vi "20211022_HW02.vi"() -> ()   [LabVIEW 2019]
panel:
  out "Result":string
  in  "N5":i32
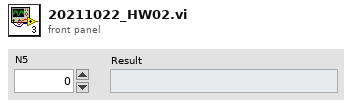
[diagram p1: front panel]
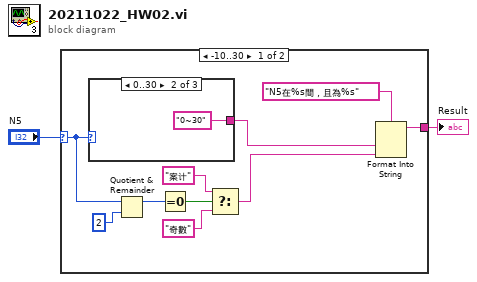
[diagram p0: block diagram]
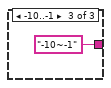
[diagram p3: hidden frame]
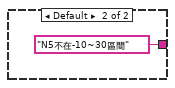
[diagram p4: hidden frame]
diagram:
  n1 = case shown="-10..30" "N5" {
    selector: "N5" -> [w12 _]
    tunnel: [w3 "N5不在-10~30區間"] -> w1
    frame -10..30 {
      n2 = case shown="0..30" w12 {
        tunnel: [_ "0~30" "-10~-1"] -> w5
        frame Default {
        }
        frame 0..30 {
        }
        frame -10..-1 {
        }
      }
      n3 = Quotient & Remainder(x=w12, y=2) -> (x-y*floor(x/y)=w10:i32)  [unwired: 1 out]
      n4 = Equal To 0?(x=w10) -> (x = 0?=w9:bool)
      n5 = Select(t="案计", s=w9, f="奇數") -> (s? t:f=w4:string)
      n6 = Format Into String(format string="N5在%s間，且為%s", w5, w4) -> (resulting string=w3:string)  [unwired: 2 in, 1 out]
    }
    frame Default {
    }
  }
  "Result" <- w1
